vi "(BASVR) AVS Noise.vi"(9 "AVS Input":T1) -> (1 "ADC 2":i32, 2 "Resistance":sgl, 3 "AVS Output":T1)   [LabVIEW 2023]
uses:
  <vilib>/numeric/Random Number (Range) U64.vi
  <vilib>/numeric/Random Number (Range) DBL.vi
  <vilib>/numeric/Random Number (Range) I64.vi
  <vilib>/numeric/sub_Random U32.vi
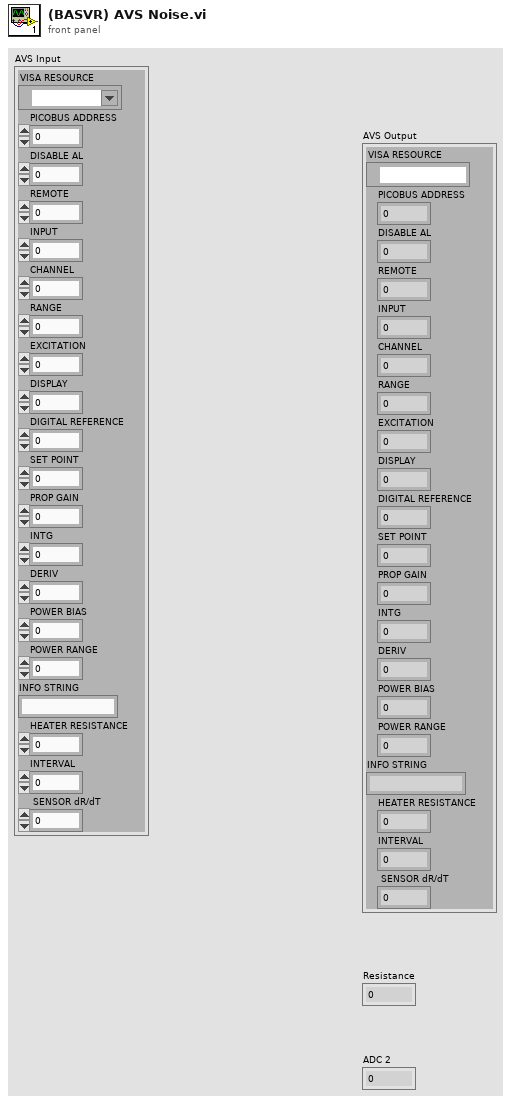
[diagram p1: front panel]
types:
  T1 = cluster{"VISA RESOURCE":refnum<visa-resource-name>, "PICOBUS ADDRESS":u8, "DISABLE AL":u8, "REMOTE":u8, "INPUT":u8, "CHANNEL":u8, "RANGE":u8, "EXCITATION":u8, "DISPLAY":u8, "DIGITAL REFERENCE":u16, "SET POINT":dbl, "PROP GAIN":u8, "INTG":u8, "DERIV":u8, "POWER BIAS":u8, "POWER RANGE":u8, "INFO STRING":string, "HEATER RESISTANCE":dbl, "INTERVAL":u8, " SENSOR dR/dT":u8}
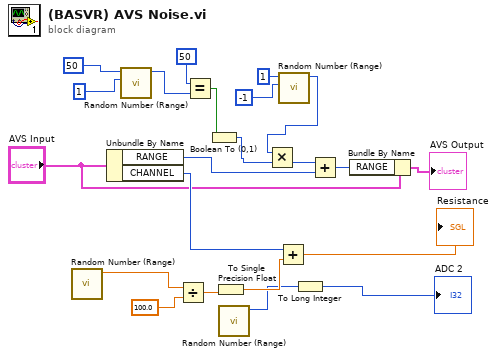
[diagram p0: block diagram]
diagram:
  n1 = call-poly <vilib>:"Random Number (Range).vi"() -> ("number"=w19:dbl)  [unwired: 11 in]
  n2 = Unbundle By Name("AVS Input") -> ("RANGE"=w9:u8, "CHANNEL"=w15:u8)
  n3 = call-poly <vilib>:"Random Number (Range).vi"("lower bound (-100)"=i64 1, "upper bound (100)"=i64 50) -> ("number"=w12:i64)  [unwired: 9 in]
  n4 = Divide(x=w19, y=100.0) -> (x/y=w21:dbl)
  n5 = Equal?(x=i64 50, y=w12) -> (x = y?=w10:bool)
  n6 = Boolean To (0,1)(Boolean=w10) -> (0, 1=w8:i16)
  n7 = To Single Precision Float(number=w21) -> (single precision float=w22:sgl)
  n8 = call-poly <vilib>:"Random Number (Range).vi"() -> ("number"=w16:u64)  [unwired: 11 in]
  n9 = Add(x=w15, y=w22) -> (x+y=→"Resistance":sgl)
  n10 = call-poly <vilib>:"Random Number (Range).vi"("lower bound (-100)"=i64 -1, "upper bound (100)"=i64 1) -> ("number"=w1:i64)  [unwired: 9 in]
  n11 = Multiply(x=w1, y=w8) -> (x*y=w2:i64)
  n12 = To Long Integer(number=w16) -> (32bit integer=→"ADC 2":i32)
  n13 = Add(x=w2, y=w9) -> (x+y=w3:i64)
  n14 = Bundle By Name(cluster="AVS Input", "RANGE"=w3) -> (→"AVS Output":T1)
